vi "Destroy User Events.vi"(8 "error in (no error)":errorcluster, 11 "GUI in":refnum<class "GUI.lvclass">) -> (0 "error out":errorcluster, 3 "GUI out":refnum<class "GUI.lvclass">)   [LabVIEW 2020, in "GUI.lvlib" / "GUI.lvclass"]
uses:
  GUI.lvclass
  GUI.lvclass/GUI.ctl
  <vilib>/Utility/config.llb/NI_LVConfig.lvlib
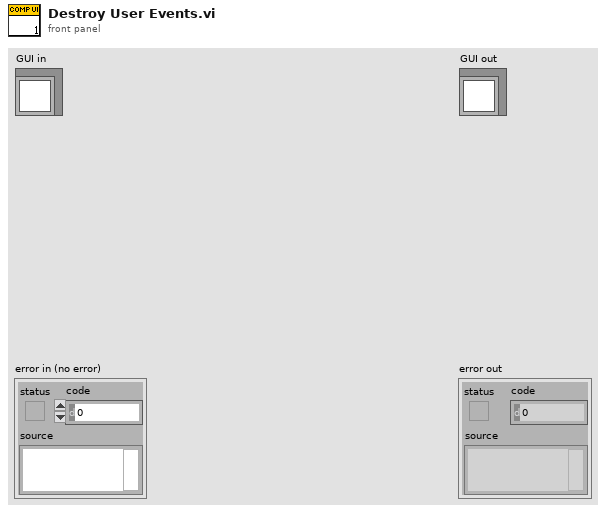
[diagram p1: front panel]
types:
  T1 = typedef "NI_LVConfig.lvlib/Config Data RefNum.ctl" = refnum<k1>
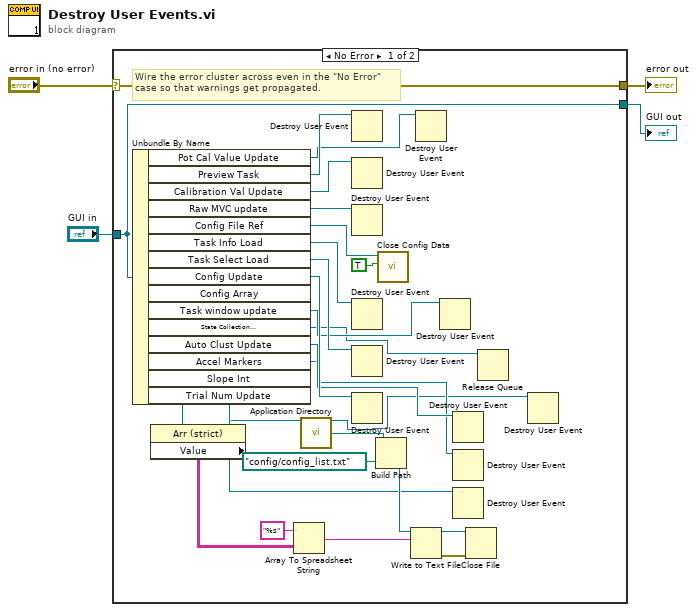
[diagram p0: block diagram]
diagram:
  n1 = case shown="No Error" "error in (no error)" {
    selector: "error in (no error)" -> [w30 w32]
    tunnel: [w30 w32] -> w3
    tunnel: [w29 w31] -> w1
    tunnel: "GUI in" -> [w29 w31]
    frame No Error {
      # "Wire the error cluster across even in the \"No Error\"\ncase so that warnings get propagated."
      n2 = Unbundle By Name(w29) -> ("Pot Cal Value Update"=w9:refnum<user-event>, "Preview Task"=w28:refnum<user-event>, "Calibration Val Update"=w27:refnum<user-event>, "Raw MVC update"=w26:refnum<user-event>, "Config File Ref"=w25:T1, "Task Info Load"=w23:refnum<user-event>, "Task Select Load"=w22:refnum<user-event>, "Config Update"=w21:refnum<user-event>, "Config Array"=w13:refnum<vi>, "Task window update"=w11:refnum<user-event>, "State Collection \nQ"=w10:refnum<queue>, "Auto Clust Update"=w8:refnum<user-event>, "Accel Markers"=w7:refnum<user-event>, "Slope Int"=w6:refnum<user-event>, "Trial Num Update"=w5:refnum<user-event>)
      n3 = property class="Arr (strict)"(reference=w13) -> ("Value"=w12:string[][])  [unwired: 1 in, 2 out]
      n4 = Array To Spreadsheet String(array=w12, 3:"%s" ("format string")) -> (spreadsheet string=w20:string)  [unwired: 1 in]
      n5 = call <vilib>:"Application Directory.vi"() -> ("Application Directory"=w19:path)
      n6 = Destroy User Event(user event=w28) -> ()  [unwired: 1 in, 1 out]
      n7 = Destroy User Event(user event=w27) -> ()  [unwired: 1 in, 1 out]
      n8 = Destroy User Event(user event=w26) -> ()  [unwired: 1 in, 1 out]
      n9 = Destroy User Event(user event=w23) -> ()  [unwired: 1 in, 1 out]
      n10 = Destroy User Event(user event=w22) -> ()  [unwired: 1 in, 1 out]
      n11 = Destroy User Event(user event=w21) -> ()  [unwired: 1 in, 1 out]
      n12 = Build Path(base path=w19, name or relative path=path "config/config_list.txt") -> (appended path=w14:path)
      n13 = call <vilib>:"Close Config Data.vi"("write file if changed (T)"=TRUE, "refnum"=w25) -> ()  [unwired: 8 in, 2 out]
      n14 = Write to Text File(file (use dialog)=w14, text=w20) -> (refnum out=w16:refnum<file>, error out=w15:errorcluster)  [unwired: 2 in, 1 out]
      n15 = Destroy User Event(user event=w9) -> ()  [unwired: 1 in, 1 out]
      n16 = Destroy User Event(user event=w11) -> ()  [unwired: 1 in, 1 out]
      n17 = Destroy User Event(user event=w8) -> ()  [unwired: 1 in, 1 out]
      n18 = Destroy User Event(user event=w7) -> ()  [unwired: 1 in, 1 out]
      n19 = Destroy User Event(user event=w6) -> ()  [unwired: 1 in, 1 out]
      n20 = Close File(refnum=w16, error in=w15) -> ()  [unwired: 2 out]
      n21 = Release Queue(queue=w10) -> ()  [unwired: 2 in, 3 out]
      n22 = Destroy User Event(user event=w5) -> ()  [unwired: 1 in, 1 out]
    }
    frame Error {
    }
  }
  "error out" <- w3
  "GUI out" <- w1
